vi "Update PartsMeasurementsMaping.vi"(0 "InspectionMcId":string, 1 "NewLSL":dbl, 2 "NewUSL":dbl, 3 "NewNominalValue":dbl, 5 "PartName":string, 7 "MeasurementName":string, 9 "Status1":bool, 11 "error in":errorcluster, 12 "NewLCL":dbl, 13 "NewUCL":dbl) -> (4 "Status":string, 15 "error out":errorcluster)   [LabVIEW 2019, in "DataLogger.lvclass"]
uses:
  DataLogger.lvclass
  <vilib>/httpClient/LabVIEWHTTPClient.lvlib
  <vilib>/httpClient/POSTBuffer.vi
panel:
  out "headers":string
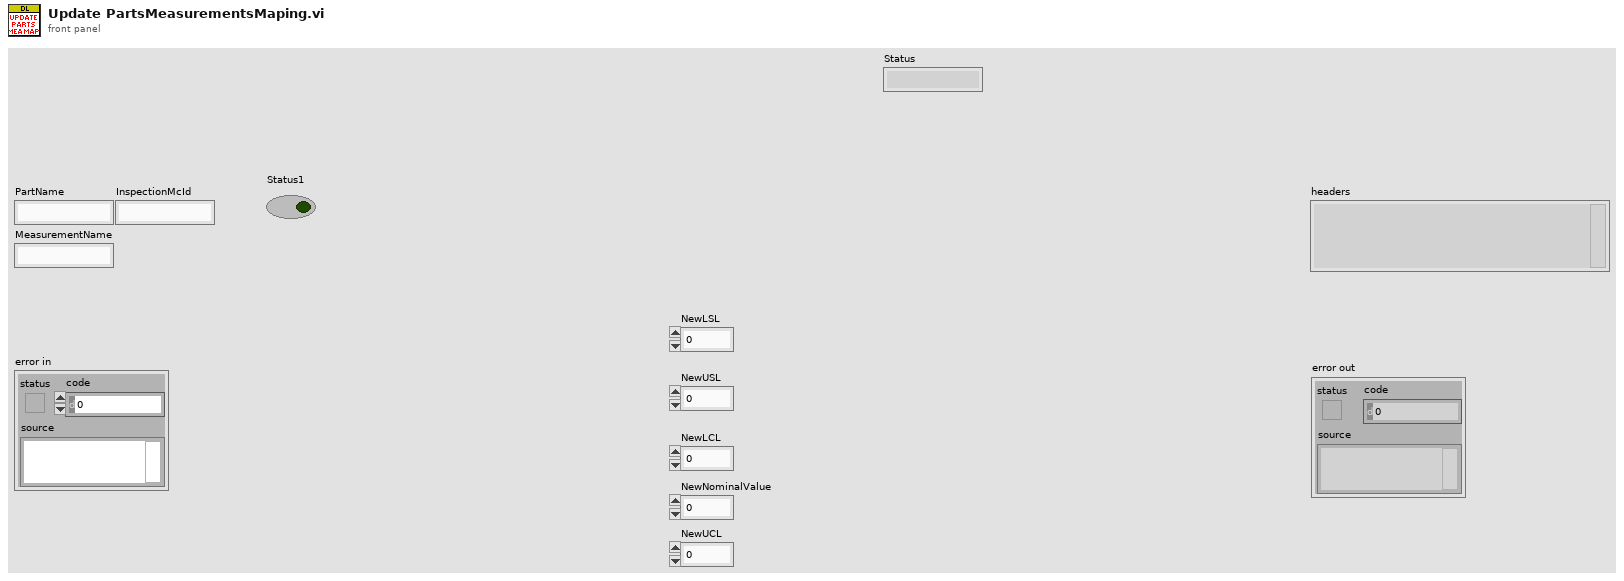
[diagram p1: front panel]
types:
  T1 = typedef "LabVIEWHTTPClient.lvlib/ClientHandle.ctl" = refnum<k1>
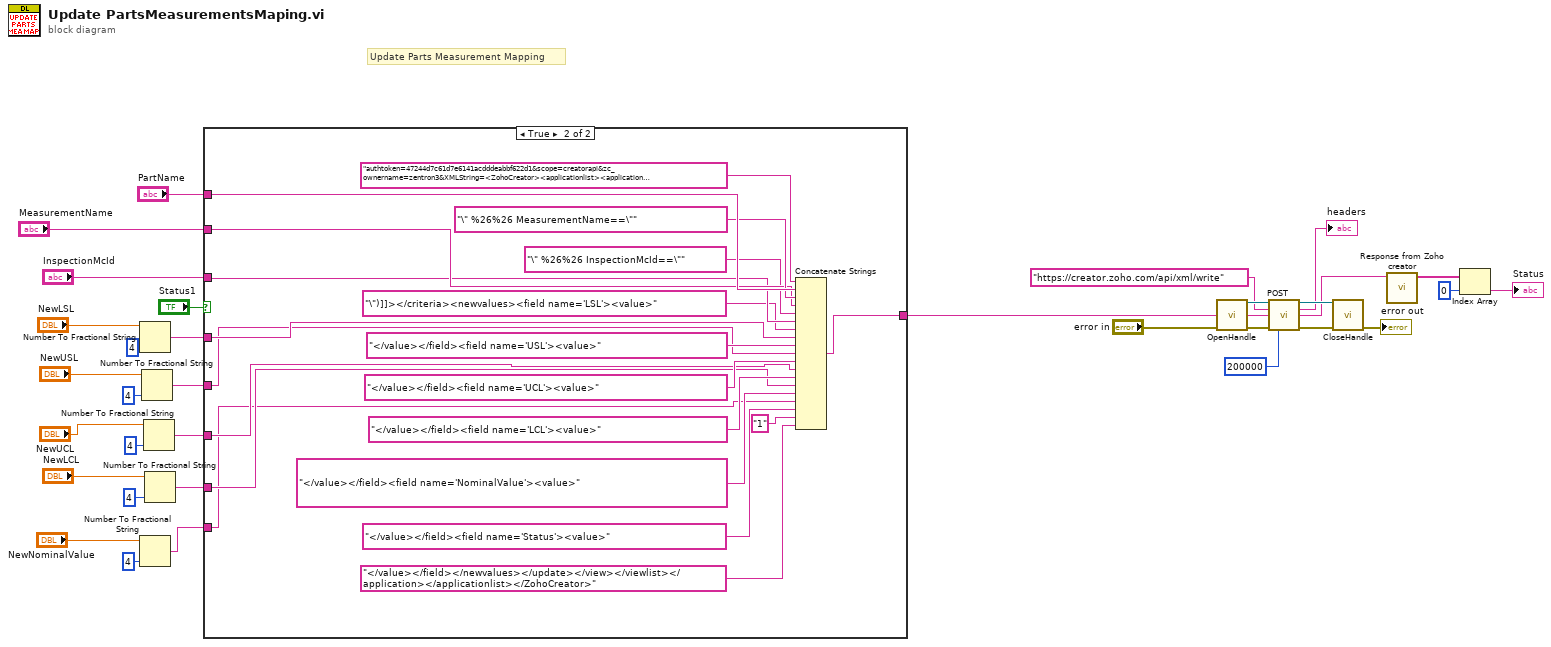
[diagram p0: block diagram]
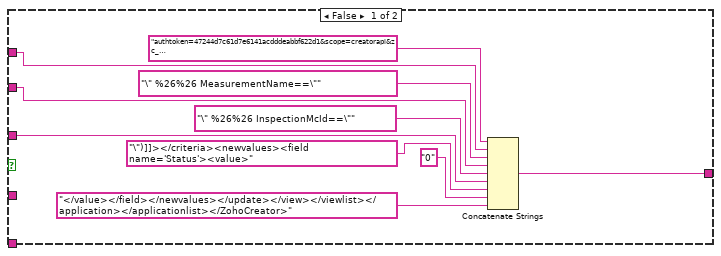
[diagram p2: hidden frame]
diagram:
  # "Update Parts Measurement Mapping"
  n1 = Number To Fractional String(number="NewLSL", precision (6)=i16 4) -> (F-format string=w10:string)  [unwired: 2 in]
  n2 = Number To Fractional String(number="NewNominalValue", precision (6)=i16 4) -> (F-format string=w6:string)  [unwired: 2 in]
  n3 = Number To Fractional String(number="NewUSL", precision (6)=i16 4) -> (F-format string=w9:string)  [unwired: 2 in]
  n4 = Number To Fractional String(number="NewUCL", precision (6)=i16 4) -> (F-format string=w8:string)  [unwired: 2 in]
  n5 = Number To Fractional String(number="NewLCL", precision (6)=i16 4) -> (F-format string=w7:string)  [unwired: 2 in]
  n6 = case shown="True" "Status1" {
    tunnel: "PartName" -> [w35 w62]
    tunnel: "MeasurementName" -> [w36 w60]
    tunnel: "InspectionMcId" -> [w34 w58]
    tunnel: [w38 w50] -> w28
    tunnel: w10 -> [_ w48]
    tunnel: w9 -> [_ w47]
    tunnel: w8 -> [_ w46]
    tunnel: w7 -> [_ w45]
    tunnel: w6 -> [_ w44]
    frame False {
      n7 = Concatenate Strings("authtoken=47244d7c61d7e6141acdddeabbf622d1&scope=creatorapi&zc_ownername=zentron3&XMLString=<ZohoCreator><applicationlist><application name='iiot-gtron'><viewlist><view name='SimulatedPartsMeasurementsMApping_Report'><update><criteria><![CDATA[(PartName==\"" ("string"), w35, "\" %26%26 MeasurementName==\"" ("string"), w36, "\" %26%26 InspectionMcId==\"" ("string"), w34, "\")]]></criteria><newvalues><field name='Status'><value>" ("string"), "0" ("string"), "</value></field></newvalues></update></view></viewlist></application></applicationlist></ZohoCreator>" ("string")) -> (w38:string)
    }
    frame True {
      n8 = Concatenate Strings("authtoken=47244d7c61d7e6141acdddeabbf622d1&scope=creatorapi&zc_ownername=zentron3&XMLString=<ZohoCreator><applicationlist><application name='iiot-gtron'><viewlist><view name='SimulatedPartsMeasurementsMApping_Report'><update><criteria><![CDATA[(PartName==\"" ("string"), w62, "\" %26%26 MeasurementName==\"" ("string"), w60, "\" %26%26 InspectionMcId==\"" ("string"), w58, "\")]]></criteria><newvalues><field name='LSL'><value>" ("string"), w48, "</value></field><field name='USL'><value>" ("string"), w47, "</value></field><field name='UCL'><value>" ("string"), w46, "</value></field><field name='LCL'><value>" ("string"), w45, "</value></field><field name='NominalValue'><value>" ("string"), w44, "</value></field><field name='Status'><value>" ("string"), "1" ("string"), "</value></field></newvalues></update></view></viewlist></application></applicationlist></ZohoCreator>" ("string")) -> (w50:string)
    }
  }
  n9 = call <vilib>:"OpenHandle.vi"("error in (no error)"="error in") -> ("client handle out"=w30:T1, "error out"=w24:errorcluster)  [unwired: 13 in]
  n10 = call-poly <vilib>:"POST.vi"("client handle"=w30, "url"="https://creator.zoho.com/api/xml/write", "buffer"=w28, "error in (no error)"=w24, "timeout (10000)"=200000) -> ("client handle out"=w29:T1, "headers"=→"headers":string, "body"=w5:string, "error out"=w23:errorcluster)  [unwired: 7 in]
  n11 = call <vilib>:"CloseHandle.vi"("client handle"=w29, "error in (no error)"=w23) -> ("error out"=→"error out":errorcluster)  [unwired: 13 in]
  n12 = call "Response from Zoho creator.vi"("body"=w5) -> ("decimated array"=w4:string[])  [unwired: 9 in, 1 out]
  n13 = Index Array(array=w4, index=0) -> (element=→"Status":string)
